vi "readFromXML.vi"(8 "error in (no error)":errorcluster, 10 "XML in":string="<scientTargetAbsorbOffset>\n  <num2>Both</num2>\n</scientTargetAbsorbOffset>", 11 "AbsorbOffset in":refnum<class "AbsorbOffset.lvclass">) -> (0 "error out":errorcluster, 3 "AbsorbOffset out":refnum<class "AbsorbOffset.lvclass">)   [LabVIEW 2014, in "TCSDataDefinitions.lvlib" / "TCSCommand.lvlib" / "OffsetCommands.lvlib" / "AbsorbOffset.lvclass"]
uses:
  AbsorbOffset.lvclass
  Enumerations/Num2Types.ctl
  AbsorbOffset.lvclass/AbsorbOffset.ctl
  TargetOffsetCommands/TargetOffsetCommands.lvclass
  <userlib>/Common/XML/XMLParser/XMLParser.lvclass
  OffsetCommands.lvlib
panel:
  out "num2":T1=enum."Both"
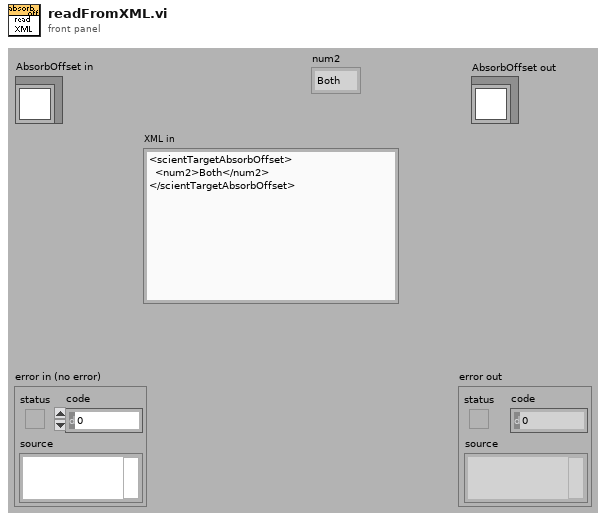
[diagram p1: front panel]
types:
  T1 = typedef "TCSDataDefinitions.lvlib/TCSCommand.lvlib/OffsetCommands.lvlib/Num2Types.ctl" = enum16{"User", "Handset", "Both"}
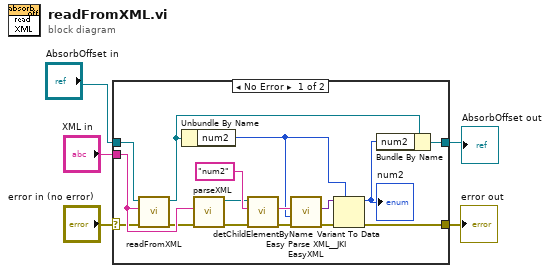
[diagram p0: block diagram]
diagram:
  n1 = case shown="No Error" "error in (no error)" {
    selector: "error in (no error)" -> [w15 w23]
    tunnel: [w7 w23] -> w4
    tunnel: [w19 w22] -> w2
    tunnel: "AbsorbOffset in" -> [w18 w22]
    tunnel: "XML in" -> [w16 _]
    frame No Error {
      n2 = call-parent "readFromXML.vi"("error in (no error)"=w15, "XML in"=w16, "TargetOffsetCommands in"=w18) -> ("error out"=w14:errorcluster, "TargetOffsetCommands out"=w17:refnum<class "AbsorbOffset.lvclass">)  [unwired: 7 out]
      n3 = Unbundle By Name(w17) -> ("num2"=w9:T1)
      n4 = call <userlib>:"parseXML.vi"("error in (no error)"=w14, "XMLString in"=w16) -> ("error out"=w21:errorcluster, "Element out"=w6:refnum<class "XMLParser.lvclass">)  [unwired: 8 in]
      n5 = call <userlib>:"detChildElementByName.vi"("error in (no error)"=w21, "childName"="num2" ("Num2"), "Element in"=w6) -> ("error out"=w10:errorcluster, "childXML"=w11:string)  [unwired: 5 in, 2 out]
      n6 = call <vilib>:"Easy Parse XML__JKI EasyXML.vi"("error in (no error)"=w10, "LabVIEW Data (Type)"=w9, "XML String"=w11) -> ("error out"=w13:errorcluster, "LabVIEW Data"=w12:variant)  [unwired: 7 in]
      n7 = Variant To Data(error in=w13, type=w9, Variant=w12) -> (data=w8:T1, error out=w7:errorcluster)
      "num2" <- w8
      n8 = Bundle By Name(cluster=w17, "num2"=w8) -> (w19:refnum<class "AbsorbOffset.lvclass">)
    }
    frame Error {
    }
  }
  "error out" <- w4
  "AbsorbOffset out" <- w2
